vi "CheckLimitsBrasse.vi"(8 "Z-Axis Field (kG)":dbl, 11 "Y-Axis Field (kG)":dbl) -> (0 "Within Limit":bool)   [LabVIEW 2009]
panel:
  out "Z-Limit":dbl
  in  "Allowed Magnet Vectors Z-Axis":dbl[](array[numeric])=[90.0, 80.0, 70.0, 60.0, 50.0, 40.0, 0.0]
  in  "Allowed Magnet Vectors Y-Axis":dbl[](array[numeric])=[0.0, 15.0, 20.0, 25.0, 30.0, 40.0, 45.0]
  out "Bereich":u16(ring) items=["0<By<15", "15<By<20", "20<By<25", "25<By<30", "30<By<40", "40<By<45"]
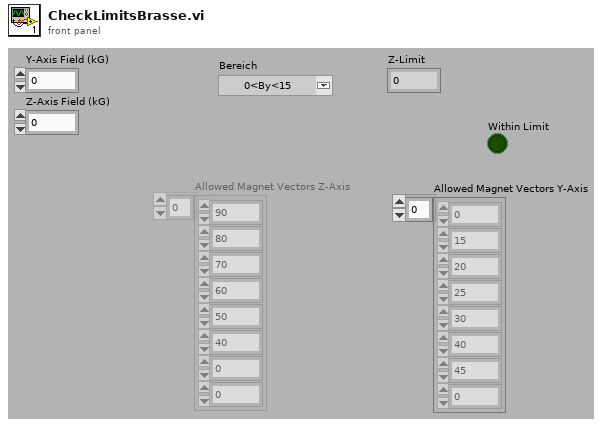
[diagram p1: front panel]
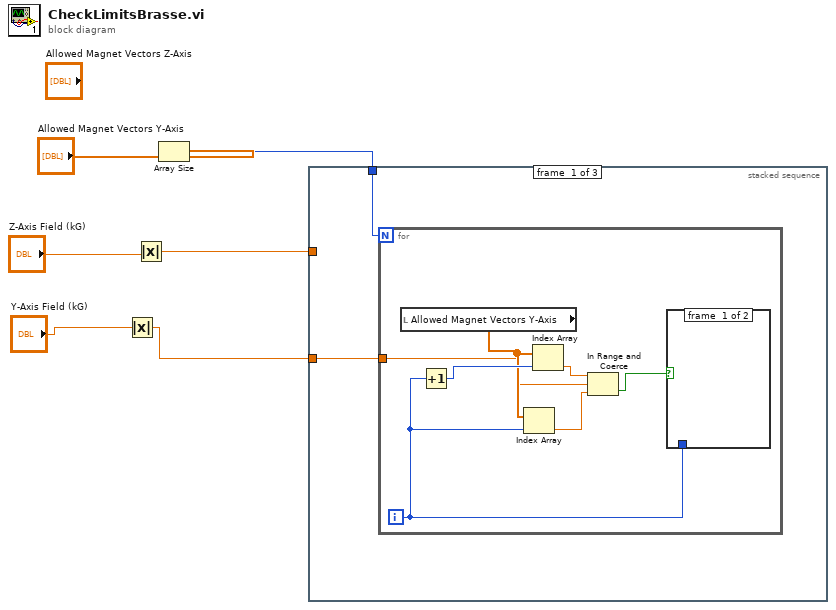
[diagram p0: block diagram]
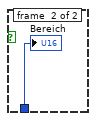
[diagram p2: hidden frame]
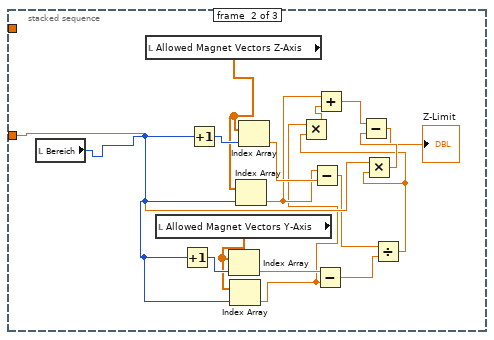
[diagram p3: hidden frame]
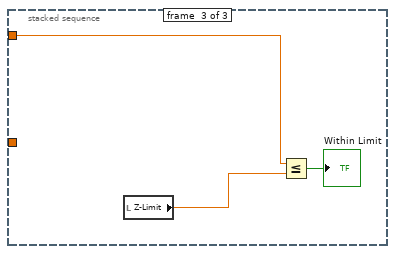
[diagram p4: hidden frame]
diagram:
  n1 = Absolute Value(x="Y-Axis Field (kG)") -> (abs(x)=w2:dbl)
  n2 = Absolute Value(x="Z-Axis Field (kG)") -> (abs(x)=w1:dbl)
  n3 = Array Size(array="Allowed Magnet Vectors Y-Axis") -> (size(s)=w3:i32)
  n4 = stacked-sequence {
    tunnel: w3 -> [w8 _ _]
    tunnel: w2 -> [w7 w32 _]
    tunnel: w1 -> [_ _ w35]
    frame #0 {
      n5 = for {
        N: w8 -> [_]
        tunnel: w7 -> [w11]
        i -> [w9]
        n6 = local read "Allowed Magnet Vectors Y-Axis"() -> (w14:dbl[])
        n7 = Increment(x=w9) -> (x+1=w15:i32)
        n8 = Index Array(array=w14, index=w9) -> (element=w13:dbl)
        n9 = Index Array(array=w14, index=w15) -> (element=w12:dbl)
        n10 = In Range and Coerce(upper limit=w12, x=w11, lower limit=w13) -> (In Range?=w10:bool)  [unwired: 1 out]
        n11 = case shown="False" w10 {
          tunnel: w9 -> [_ w16]
          frame #0 {
          }
          frame #1 {
            "Bereich" <- w16
          }
        }
      }
    }
    frame #1 {
      n12 = local read "Bereich"() -> (w33:u16)
      n13 = local read "Allowed Magnet Vectors Z-Axis"() -> (w30:dbl[])
      n14 = local read "Allowed Magnet Vectors Y-Axis"() -> (w25:dbl[])
      n15 = Increment(x=w33) -> (x+1=w26:u16)
      n16 = Increment(x=w33) -> (x+1=w31:u16)
      n17 = Index Array(array=w25, index=w26) -> (element=w24:dbl)
      n18 = Index Array(array=w25, index=w33) -> (element=w19:dbl)
      n19 = Index Array(array=w30, index=w33) -> (element=w21:dbl)
      n20 = Index Array(array=w30, index=w31) -> (element=w29:dbl)
      n21 = Subtract(x=w21, y=w29) -> (x-y=w23:dbl)
      n22 = Subtract(x=w24, y=w19) -> (x-y=w22:dbl)
      n23 = Divide(x=w23, y=w22) -> (x/y=w20:dbl)
      n24 = Multiply(x=w19, y=w20) -> (x*y=w18:dbl)
      n25 = Add(x=w21, y=w18) -> (x+y=w17:dbl)
      n26 = Multiply(x=w32, y=w20) -> (x*y=w28:dbl)
      n27 = Subtract(x=w17, y=w28) -> (x-y=→"Z-Limit":dbl)
    }
    frame #2 {
      n28 = local read "Z-Limit"() -> (w36:dbl)
      n29 = Less Or Equal?(x=w35, y=w36) -> (x <= y?=→"Within Limit":bool)
    }
  }
